vi "create_i.vi"(10 "Lorentzian Width":dbl, 11 "Numeric":dbl) -> (3 "Numeric 2":dbl)   [LabVIEW 2018]
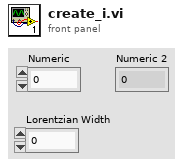
[diagram p1: front panel]
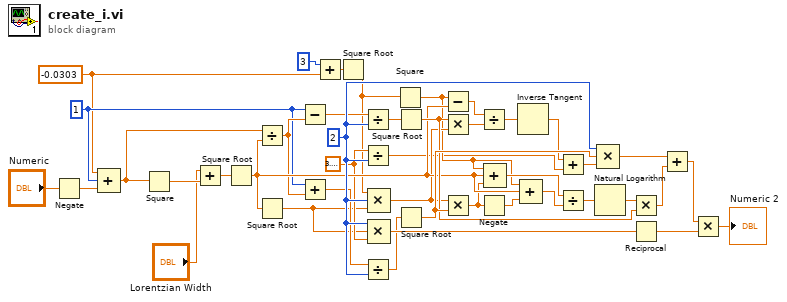
[diagram p0: block diagram]
diagram:
  w19 = 3.141592653589793
  w36 = 2
  w16 = 1
  w13 = -0.0303
  n1 = Negate(x="Numeric") -> (-x=w1:dbl)
  n2 = Compound Arithmetic op=ADD(w13, w16, w1) -> (w9:dbl)
  n3 = Square(x=w9) -> (x^2=w7:dbl)
  n4 = Add(x="Lorentzian Width", y=w7) -> (x+y=w8:dbl)
  n5 = Square Root(x=w8) -> (sqrt(x)=w30:dbl)
  n6 = Divide(x=w9, y=w30) -> (x/y=w17:dbl)
  n7 = Square Root(x=w30) -> (sqrt(x)=w2:dbl)
  n8 = Subtract(x=w16, y=w17) -> (x-y=w11:dbl)
  n9 = Add(x=w16, y=w17) -> (x+y=w10:dbl)
  n10 = Add(x=3, y=w13) -> (x+y=w20:dbl)
  n11 = Square Root(x=w20) -> (sqrt(x)=w4:dbl)
  n12 = Divide(x=w11, y=w36) -> (x/y=w15:dbl)
  n13 = Divide(x=w19, y=w36) -> (x/y=w25:dbl)
  n14 = Divide(x=w10, y=w36) -> (x/y=w14:dbl)
  n15 = Compound Arithmetic op=MULTIPLY(w4, w36, w2) -> (w28:dbl)
  n16 = Compound Arithmetic op=MULTIPLY(w36, w2, w19) -> (w18:dbl)
  n17 = Square(x=w4) -> (x^2=w27:dbl)
  n18 = Square Root(x=w15) -> (sqrt(x)=w35:dbl)
  n19 = Square Root(x=w14) -> (sqrt(x)=w37:dbl)
  n20 = Subtract(x=w27, y=w30) -> (x-y=w21:dbl)
  n21 = Multiply(x=w35, y=w28) -> (x*y=w22:dbl)
  n22 = Multiply(x=w28, y=w37) -> (x*y=w29:dbl)
  n23 = Divide(x=w21, y=w22) -> (x/y=w23:dbl)
  n24 = Negate(x=w29) -> (-x=w26:dbl)
  n25 = Compound Arithmetic op=ADD(w27, w30, w29) -> (w31:dbl)
  n26 = Inverse Tangent(1:w23) -> (0:w24:dbl)
  n27 = Compound Arithmetic op=ADD(w27, w30, w26) -> (w32:dbl)
  n28 = Add(x=w24, y=w25) -> (x+y=w38:dbl)
  n29 = Divide(x=w31, y=w32) -> (x/y=w33:dbl)
  n30 = Natural Logarithm(1:w33) -> (0:w34:dbl)
  n31 = Compound Arithmetic op=MULTIPLY(w36, w37, w38) -> (w39:dbl)
  n32 = Multiply(x=w34, y=w35) -> (x*y=w40:dbl)
  n33 = Reciprocal(x=w18) -> (1/x=w42:dbl)
  n34 = Add(x=w39, y=w40) -> (x+y=w41:dbl)
  n35 = Multiply(x=w41, y=w42) -> (x*y=→"Numeric 2":dbl)
